vi "Query Multi Eval Meas Trigger Source Catalog.vi"(8 "error in (no error)":errorcluster, 10 "Instance (1)":T1=1, 11 "VISA resource name":refnum<visa-resource-name>) -> (0 "error out":errorcluster, 2 "Trigger Source Catalog":string[](array[string]), 3 "VISA resource name out":refnum<visa-resource-name>)   [LabVIEW 2015, in "Rohde&Schwarz CMXP NR FR2 Measurement.lvlib"]
doc: "Lists all trigger source values that can be set using TRIGger:NRMMw:MEAS<i>:MEValuation:SOURce. Comma-separated list of all supported values, one string per value.\n\nAttribute:\nRSCMXPNRFR2M_ATTR_MULTI_EVAL_MEASUREMENT_TRIGGER_SOURCE_CATALOG\n\nRemote-control command:\nTRIGger:NRMMw:MEAS<i>:MEValuation:CATalog:SOURce?"
uses:
  <instrlib>/Rohde&Schwarz CMXP NR FR2 Measurement/Rohde&Schwarz CMXP NR FR2 Measurement.lvlib
  <instrlib>/Rohde&Schwarz CMXP NR FR2 Measurement/Private/_Instance.ctl
  <instrlib>/Rohde&Schwarz CMXP NR FR2 Measurement/Private/rsidr_core.llb/rsidr_core.lvlib
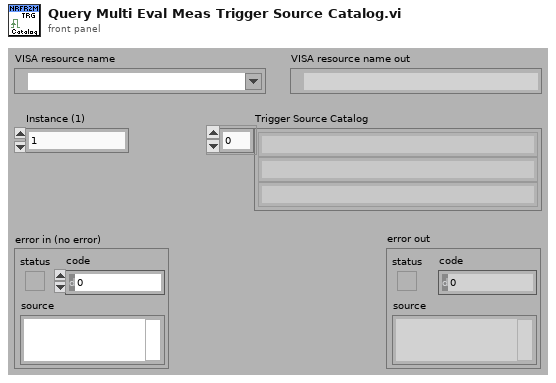
[diagram p1: front panel]
types:
  T1 = typedef "Rohde&Schwarz CMXP NR FR2 Measurement.lvlib/_Instance.ctl" = i32
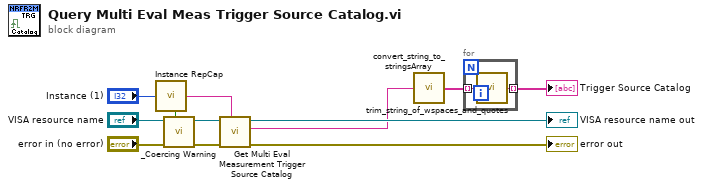
[diagram p0: block diagram]
diagram:
  n1 = call <instrlib>:"Instance RepCap.vi"("Instance In"="Instance (1)") -> ("In Range?"=w8:bool, "RepCap Identifier Out"=w7:string)  [unwired: 1 in]
  n2 = call <instrlib>:"_Coercing Warning.vi"("In Range?"=w8, "error in (no error)"="error in (no error)", "VISA resource name"="VISA resource name") -> ("error out"=w5:errorcluster, "VISA resource name out"=w6:refnum<visa-resource-name>)  [unwired: 7 in]
  n3 = call "Get Multi Eval Measurement Trigger Source Catalog"("Repeated Capabilities"=w7, "error in (no error)"=w5, "instrument handle"=w6) -> ("error out"=→"error out":errorcluster, "Multi Eval Measurement Trigger Source Catalog"=w1:string, "instrument handle out"=→"VISA resource name out":refnum<visa-resource-name>)  [unwired: 6 in]
  n4 = call <instrlib>:"convert_string_to_stringsArray.vi"("String in"=w1) -> ("string array out"=w4:string[])  [unwired: 3 in, 1 out]
  n5 = for {
    tunnel: w4 -> [w14] mode=indexing
    tunnel: [w13] -> w3 mode=indexing
    n6 = call <instrlib>:"trim_string_of_wspaces_and_quotes.vi"("String in"=w14) -> ("String out"=w13:string)  [unwired: 4 in]
  }
  "Trigger Source Catalog" <- w3
